vi "Convert State For Save.vi"(2 "Container State":T1, 3 "Display State":T2) -> (1 "Display State To Save":variant)   [LabVIEW 2018]
uses:
  Controls/State.ctl
  <vilib>/_xctls/Container State.ctl
  subvis/FP Controls.ctl
  subvis/Function Types.ctl
  Waveform Control.xctl
  <vilib>/_xctls/XControlSupport.lvlib
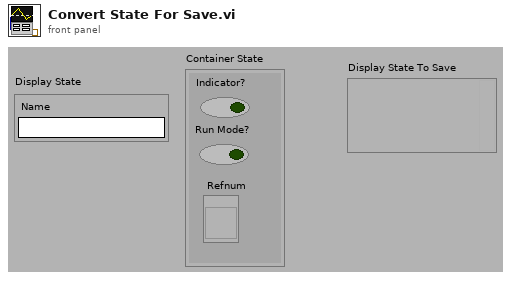
[diagram p1: front panel]
types:
  T1 = typedef "XControlSupport.lvlib/Container State.ctl" = cluster{"Indicator?":bool, "Run Mode?":bool, " Refnum":refnum<vi>}
  T2 = typedef "Waveform Control.xctl/State.ctl" = cluster{"Name":string}
  T3 = typedef "Waveform Control.xctl/FP Controls.ctl" = cluster{"Type":T4, "Periods":dbl, "Points":i32, "Offset":dbl, "Amplitdue":dbl, "Phase":dbl, "func":string}
  T4 = typedef "Waveform Control.xctl/Function Types.ctl" = enum16{"Level", "Sine", "Triangle", "Ramp", "Saw Tooth", "Square", "Function"}
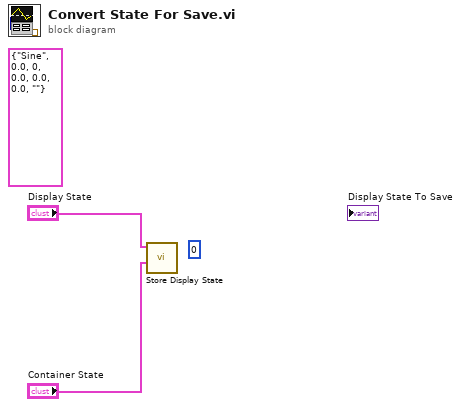
[diagram p0: block diagram]
diagram:
  (unwired) 0 ("Current Location")
  (unwired) T3 {"Type"=enum."Sine", "Periods"=0.0, "Points"=0, "Offset"=0.0, "Amplitdue"=0.0, "Phase"=0.0, "func"=""} ("Controls")
  n1 = call "Store Display State.vi"("Container State In"="Container State", "State In"="Display State") -> ()  [unwired: 4 in, 6 out]
